vi "Pre Purge API.vi"(5 "Repeats":u8, 6 "ICP1-DO Channel Names":T1, 7 "PurgeDuration (s)":dbl, 8 "error in (no error)":errorcluster, 9 "Duration (s)":dbl, 10 "GIS File Path":path, 11 "TopLevel in":refnum<class "TopLevel.lvclass">) -> (0 "error out":errorcluster, 3 "TopLevel out":refnum<class "TopLevel.lvclass">)   [LabVIEW 2022 SP3, in "TopLevel.lvclass"]
uses:
  TopLevel.lvclass
  IO/Typedefs/ICP1-D0 Channel Names.ctl
  Typedefs/API Command Cluster.ctl
  Typedefs/API Command Enum.ctl
  Typedefs/Pre Purge API Data.ctl
  IO/IO.lvclass
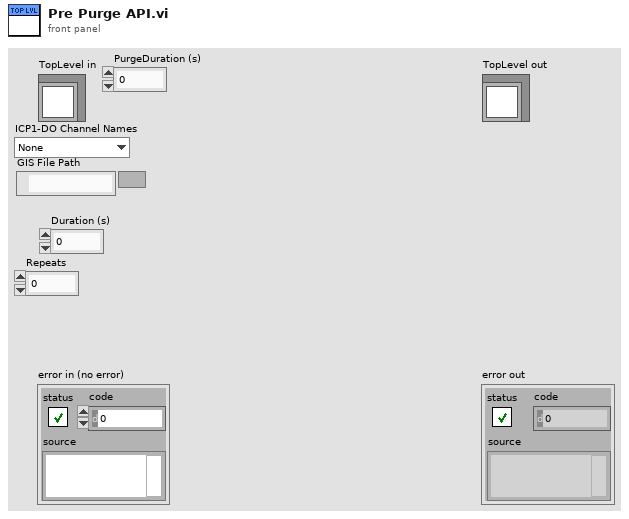
[diagram p1: front panel]
types:
  T1 = typedef "IO.lvclass/ICP1-D0 Channel Names.ctl" = enum16{"None", "Meniscus Pressure Reg PWR - R1", "Meniscus Pressure Reg PWR - R2", "Meniscus Pressure Reg PWR - R3", "Meniscus Pressure Reg PWR - R4", "Meniscus Pressure Reg PWR - R5", "Meniscus Pressure Reg PWR - R6", "Clear Stage Alarm", "Servo ON", "Purge Valve Open - R1", "Purge Valve Open - R2", "Purge Valve Open - R3", "Purge Valve Open - R4", "Purge Valve Open - R5", "Purge Valve Open - R6"}
  T2 = typedef "TopLevel.lvclass/Pre Purge API Data.ctl" = cluster{"Purge Channel Name":T1, "GIS File Path":path, "Duration (s)":dbl, "PurgeDuration (s)":dbl, "Repeats":u8}
  T3 = typedef "TopLevel.lvclass/API Command Enum.ctl" = enum16{"Execute Printer Commands", "Pre Purge", "Enable Ink Ch-1", "Enable Ink Ch-2", "Enable Ink Ch-3", "Enable Ink Ch-4", "Enable Ink Ch-5", "Enable Ink Ch-6", "Disable Ink Ch-1", "Disable Ink Ch-2", "Disable Ink Ch-3", "Disable Ink Ch-4", "Disable Ink Ch-5", "Disable Ink Ch-6", "ExecuteIdlePrintCycle", "StopIdlePrintCycle", "Abort", "LoadDLP2GUIConfig", "SaveDLP2GUIConfig", "PrimingMode", "SetHeadTemperature", "EnableHead", "EnableHeadHeat", "SetSystemMode", "HeadPrint", "AbortAll", "Send Printer String", "WriteInitXML"}
  T4 = typedef "TopLevel.lvclass/API Command Cluster.ctl" = cluster{"Command":T3, "Arguments":string, "Data":variant}
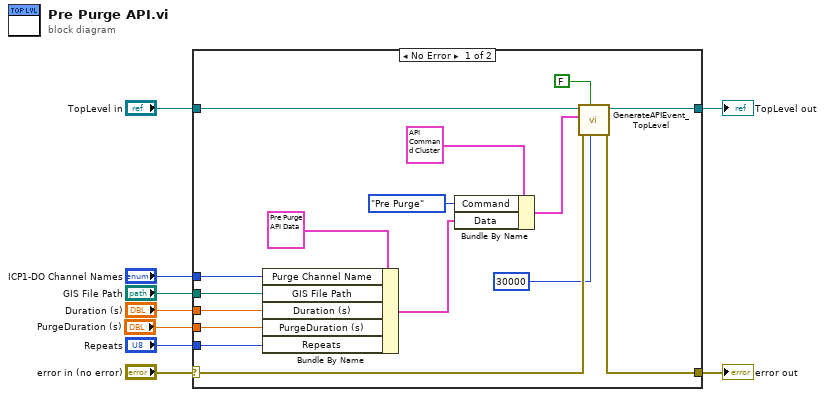
[diagram p0: block diagram]
diagram:
  n1 = case shown="No Error" "error in (no error)" {
    selector: "error in (no error)" -> [w23 w27]
    tunnel: [w22 w27] -> w8
    tunnel: [w25 w26] -> w6
    tunnel: "TopLevel in" -> [w24 w26]
    tunnel: "Duration (s)" -> [w16 _]
    tunnel: "GIS File Path" -> [w15 _]
    tunnel: "ICP1-DO Channel Names" -> [w14 _]
    tunnel: "PurgeDuration (s)" -> [w11 _]
    tunnel: "Repeats" -> [w10 _]
    frame No Error {
      n2 = Bundle By Name(cluster=T2 {"Purge Channel Name"=enum."Purge Valve Open - R1", "GIS File Path"=path "", "Duration (s)"=0.1, "PurgeDuration (s)"=0.1, "Repeats"=0} ("Pre Purge API Data"), "Purge Channel Name"=w14, "GIS File Path"=w15, "Duration (s)"=w16, "PurgeDuration (s)"=w11, "Repeats"=w10) -> (w17:T2)
      n3 = Bundle By Name(cluster=T4 {"Command"=enum."Execute Printer Commands", "Arguments"="", "Data"=variant} ("API Command Cluster"), "Command"=API_Command_Enum."Pre Purge", "Data"=w17) -> (w19:T4)
      n4 = call-dynamic "GenerateAPIEvent_TopLevel.vi"("Timeout (ms)"=u32 30000, "Wait (F)"=FALSE, "error in (no error)"=w23, "API Command Cluster"=w19, "TopLevel in"=w24) -> ("error out"=w22:errorcluster, "TopLevel out"=w25:refnum<class "TopLevel.lvclass">)  [unwired: 5 in]
    }
    frame Error {
    }
  }
  "error out" <- w8
  "TopLevel out" <- w6
